vi "LogNames.vi"() -> ()   [LabVIEW 2023]
panel:
  in  "Array":string[](array[string])
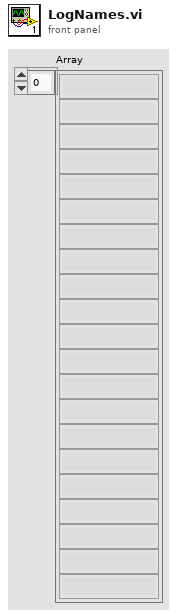
[diagram p1: front panel]
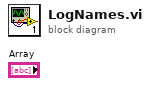
[diagram p0: block diagram]
diagram:
